vi "Remove piece.vi"(8 "error in (no error)":errorcluster, 10 "Square":T1={"File"=enum."a", "Rank"=enum."4"}, 11 "Position in":refnum<class "Position.lvclass">) -> (0 "error out":errorcluster, 1 "Removed piece":refnum<class "Piece.lvclass">, 2 "Square occupied?":bool, 3 "Position out":refnum<class "Position.lvclass">)   [LabVIEW 2016, in "Chesslib.lvlib" / "Position.lvclass"]
uses:
  Position.lvclass
  typedef/Square.ctl
  typedef/File.ctl
  typedef/Rank.ctl
  Pieces/Piece/Piece.lvclass
  Position.lvclass/Position.ctl
  Board/Board.lvclass
  Chesslib.lvlib
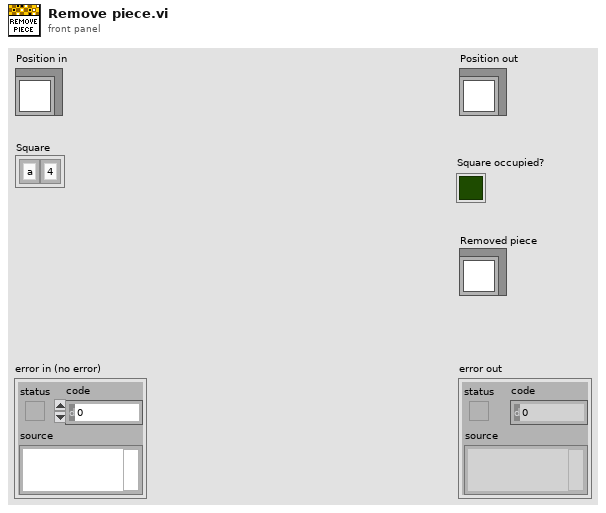
[diagram p1: front panel]
types:
  T1 = typedef "Chesslib.lvlib/Square.ctl" = cluster{"File":T2, "Rank":T3}
  T2 = typedef "Chesslib.lvlib/File.ctl" = enum8{"a", "b", "c", "d", "e", "f", "g", "h"}
  T3 = typedef "Chesslib.lvlib/Rank.ctl" = enum8{"1", "2", "3", "4", "5", "6", "7", "8"}
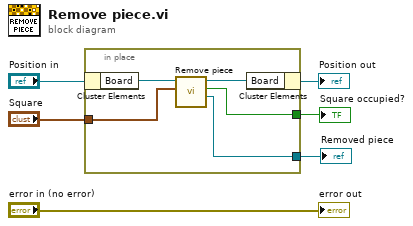
[diagram p0: block diagram]
diagram:
  n1 = in-place {
    in-place-border: "Square" -> [w9]
    in-place-border: [w8] -> w2
    in-place-border: [w7] -> w1
    n2 = in-place-cluster #1("Position in") -> ("Board"=w11:refnum<class "Board.lvclass">)
    n3 = call "Remove piece.vi"("Square"=w9, "Board in"=w11) -> ("Removed piece"=w7:refnum<class "Piece.lvclass">, "Square occupied?"=w8:bool, "Board out"=w10:refnum<class "Board.lvclass">)  [unwired: 7 in]
    n4 = in-place-cluster #1("Board"=w10) -> (→"Position out":refnum<class "Position.lvclass">)
  }
  "Removed piece" <- w1
  "Square occupied?" <- w2
  "error out" <- "error in (no error)"
